vi "Raise Abort.vi"(8 "error in (no error)":errorcluster, 11 "Guardian in":refnum<class "Guardian.lvclass">) -> (0 "error out":errorcluster, 3 "Guardian out":refnum<class "Guardian.lvclass">)   [LabVIEW 2026, in "TALOS.lvlib" / "Guardian.lvlib" / "Guardian.lvclass"]
uses:
  Guardian.lvclass
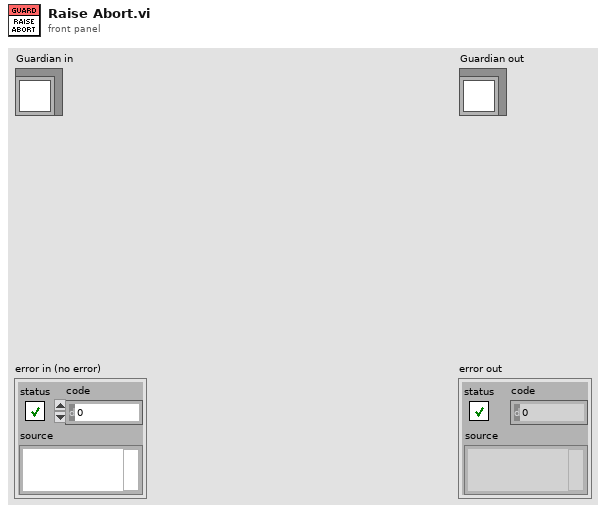
[diagram p1: front panel]
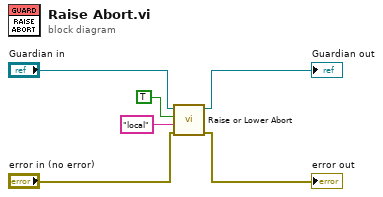
[diagram p0: block diagram]
diagram:
  n1 = call "Raise or Lower Abort.vi"("error in (no error)"="error in (no error)", "Sender"="local", "New Abort Value"=TRUE, "Guardian in"="Guardian in") -> ("error out"=→"error out":errorcluster, "Guardian out"=→"Guardian out":refnum<class "Guardian.lvclass">)  [unwired: 6 in]
